vi "Unflatten I32.vi"(3 "Flat Data":u8[](array[numeric]) format="%.0x", 4 "Endian":T1) -> (5 "I32":i32)   [LabVIEW 2021, in "DataTypes_CIF_U.lvlib"]
uses:
  Endian.ctl
  DataTypes_CIF_U.lvlib
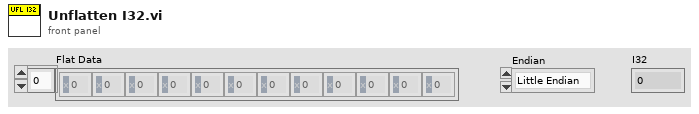
[diagram p1: front panel]
types:
  T1 = typedef "DataTypes_CIF_U.lvlib/Endian.ctl" = enum16{"Little Endian", "Big Endian"}
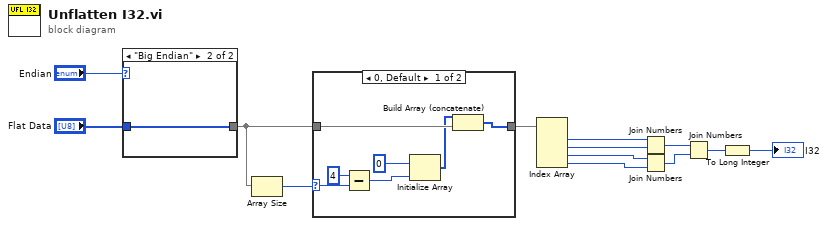
[diagram p0: block diagram]
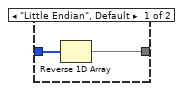
[diagram p3: hidden frame]
diagram:
  n1 = case shown="\"Big Endian\"" "Endian" {
    tunnel: "Flat Data" -> [w15 w16]
    tunnel: [w14 w16] -> w3
    frame "Little Endian", Default {
      n2 = Reverse 1D Array(array=w15) -> (reversed array=w14:u8[])
    }
    frame "Big Endian" {
    }
  }
  n3 = Array Size(array=w3) -> (size(s)=w6:i32)
  n4 = case shown="0, Default" w6 {
    selector: w6 -> [w23 _]
    tunnel: w3 -> [w19 w24]
    tunnel: [w17 w24] -> w4
    frame 0, Default {
      n5 = Subtract(x=4, y=w23) -> (x-y=w20:i32)
      n6 = Initialize Array(u8 0 ("element"), w20) -> (w18:u8[])
      n7 = Build Array (concatenate)(w18, w19) -> (w17:u8[])
    }
    frame 8.. {
    }
  }
  n8 = Index Array(array=w4) -> (element #1=w12:u8, element #2=w9:u8, element #3=w8:u8, element #4=w7:u8)  [unwired: 4 in]
  n9 = Join Numbers(hi=w12, lo=w9) -> ((hi.lo)=w11:u16)
  n10 = Join Numbers(hi=w8, lo=w7) -> ((hi.lo)=w10:u16)
  n11 = Join Numbers(hi=w11, lo=w10) -> ((hi.lo)=w1:u32)
  n12 = To Long Integer(number=w1) -> (32bit integer=→"I32":i32)
